vi "REPORT_AUDIT_DEFINE_STATUS_REAL_RESULT.vi"(9 "unit":string, 10 "max":dbl, 11 "min":dbl) -> (3 "action":T1)   [LabVIEW 2020]
uses:
  typedef/REPORT_AUDIT_define_result_audit.ctl
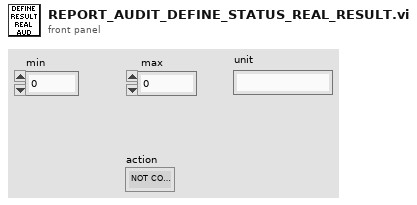
[diagram p1: front panel]
types:
  T1 = typedef "REPORT_AUDIT_define_result_audit.ctl" = enum16{"NOT CORRECT", "MIN ONLY", "MAX ONLY", "MIN AND MAX", "STATUS", "NOT CORRECT_1", "NOT CORRECT_2", "NOT CORRECT_3"}
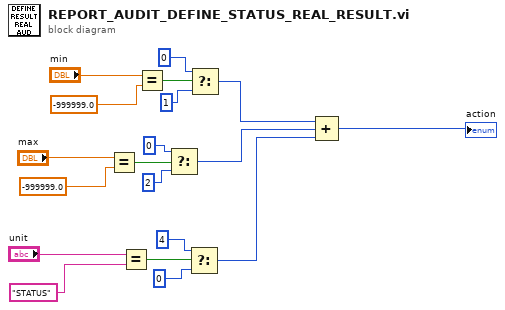
[diagram p0: block diagram]
diagram:
  n1 = Equal?(x="max", y=-999999.0) -> (x = y?=w12:bool)
  n2 = Equal?(x="unit", y="STATUS") -> (x = y?=w5:bool)
  n3 = Equal?(x="min", y=-999999.0) -> (x = y?=w15:bool)
  n4 = Select(t=u16 0, s=w12, f=u16 2) -> (s? t:f=w8:u16)
  n5 = Select(t=u16 4, s=w5, f=u16 0) -> (s? t:f=w2:u16)
  n6 = Select(t=u16 0, s=w15, f=u16 1) -> (s? t:f=w9:u16)
  n7 = Compound Arithmetic op=ADD(w9, w8, w2) -> (→"action":u16)
